vi "Generate Unique Header.vi"(8 "error in":errorcluster, 11 "TECData in":refnum<class "TECData.lvclass">) -> (0 "error out":errorcluster, 2 "Header":string[](array[string]), 3 "TECData out":refnum<class "TECData.lvclass">)   [LabVIEW 2014, in "TE Cooler.lvlib" / "TECData.lvclass"]
uses:
  TECData.lvclass
  reusable/Data/Data.lvclass/Data.ctl
  reusable/Data/Read Data ID.vi
  reusable/Data/Data.lvclass
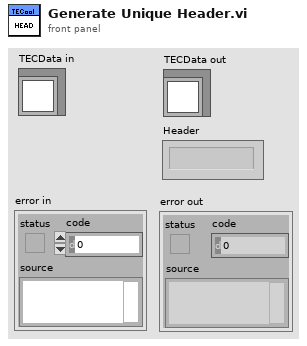
[diagram p1: front panel]
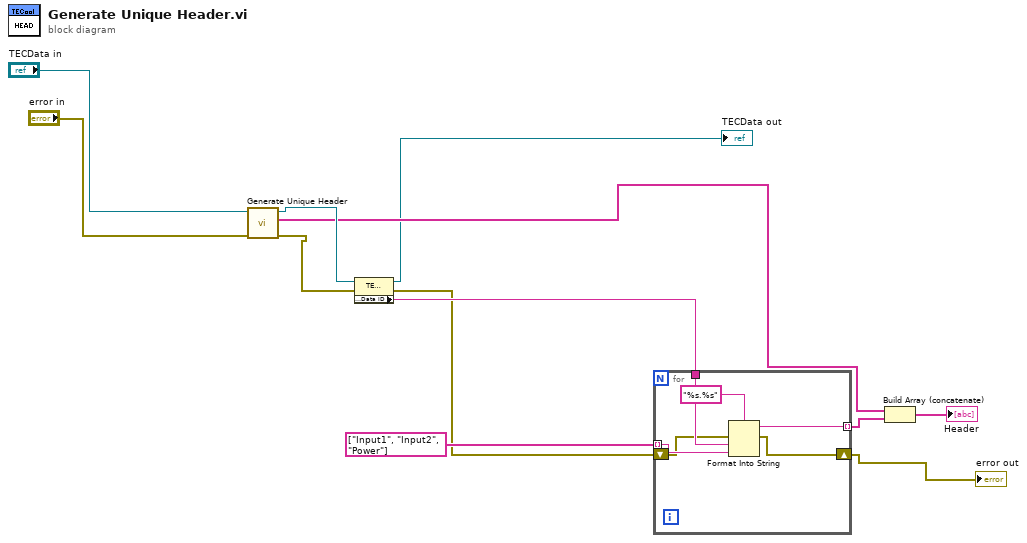
[diagram p0: block diagram]
diagram:
  n1 = call-parent "Generate Unique Header.vi"("error in"="error in", "Data in"="TECData in") -> ("error out"=w10:errorcluster, "Header"=w6:string[], "Data out"=w11:refnum<class "TECData.lvclass">)  [unwired: 7 in]
  n2 = property class="TEC Data"(reference=w11, error in=w10) -> (reference out=→"TECData out":refnum<class "TECData.lvclass">, error out=w8:errorcluster, "Accessors:Data ID"=w9:string)
  n3 = for {
    tunnel: string[] ["Input1", "Input2", "Power"] -> [w17] mode=indexing
    tunnel: w9 -> [w18]
    tunnel: [w15] -> w7 mode=indexing
    shift-right: [w14] -> w2
    shift-left: w8 -> [w13]
    n4 = Format Into String(format string="%s.%s", error in=w13, w18, w17) -> (resulting string=w15:string, error out=w14:errorcluster)  [unwired: 1 in]
  }
  "error out" <- w2
  n5 = Build Array (concatenate)(w6, w7) -> (→"Header":string[])
